vi "RunMacro_popup.vi"(0 "load?":bool, 1 "platform":u16(ring) items=["Mac", "PC"], 2 "command in":string, 3 "error in (no error)":errorcluster) -> (8 "Cancel":bool, 9 "command out":string, 10 "error out":errorcluster)   [LabVIEW 2020]
doc: "Sequence Program with the Message Handling Queue (MHQ) for the National High Magnetic Field Laboratory in Tallahassee, Florida. \nOnce you understand how the programs works, you should be able to modify this program easily. If you have any questions, contact Minseong Lee(ml10k@my.fsu.edu), who first made this program in June, 2015."
uses:
  <vilib>/Utility/file.llb/Read From Spreadsheet File (string).vi
panel:
  in  "Cancel button":bool
  in  "OK Button 2":bool
  in  "Cancel Button":bool
  in  "OK Button":bool
  out "Buffer Edit":string[](array[string])=["Wait for 1 s", "Wait for 2 s", "Wait for 1.1 s", "Wait for 1.2 s"]
  out "Path":path=path "C:/Users/shared/Sequences/MPMS_LCR_Tsweep.vi.txt"
  out "Buffer History":string[](array[string])
  in  "New Button":bool caption="New"
  in  "Commands":string(tree)="Wait for"
  in  "Sequence":i32[](listbox)=[4]
  in  "Save Button":bool caption="Save"
  in  "Save As Button":bool caption="Save As"
  out "Cursor Position":i32=4
  in  "Open Button":bool caption="Open"
  # "(1) Make a new or edit an existing sequence\n(2) Sequence must be saved\nNesting is allowed."
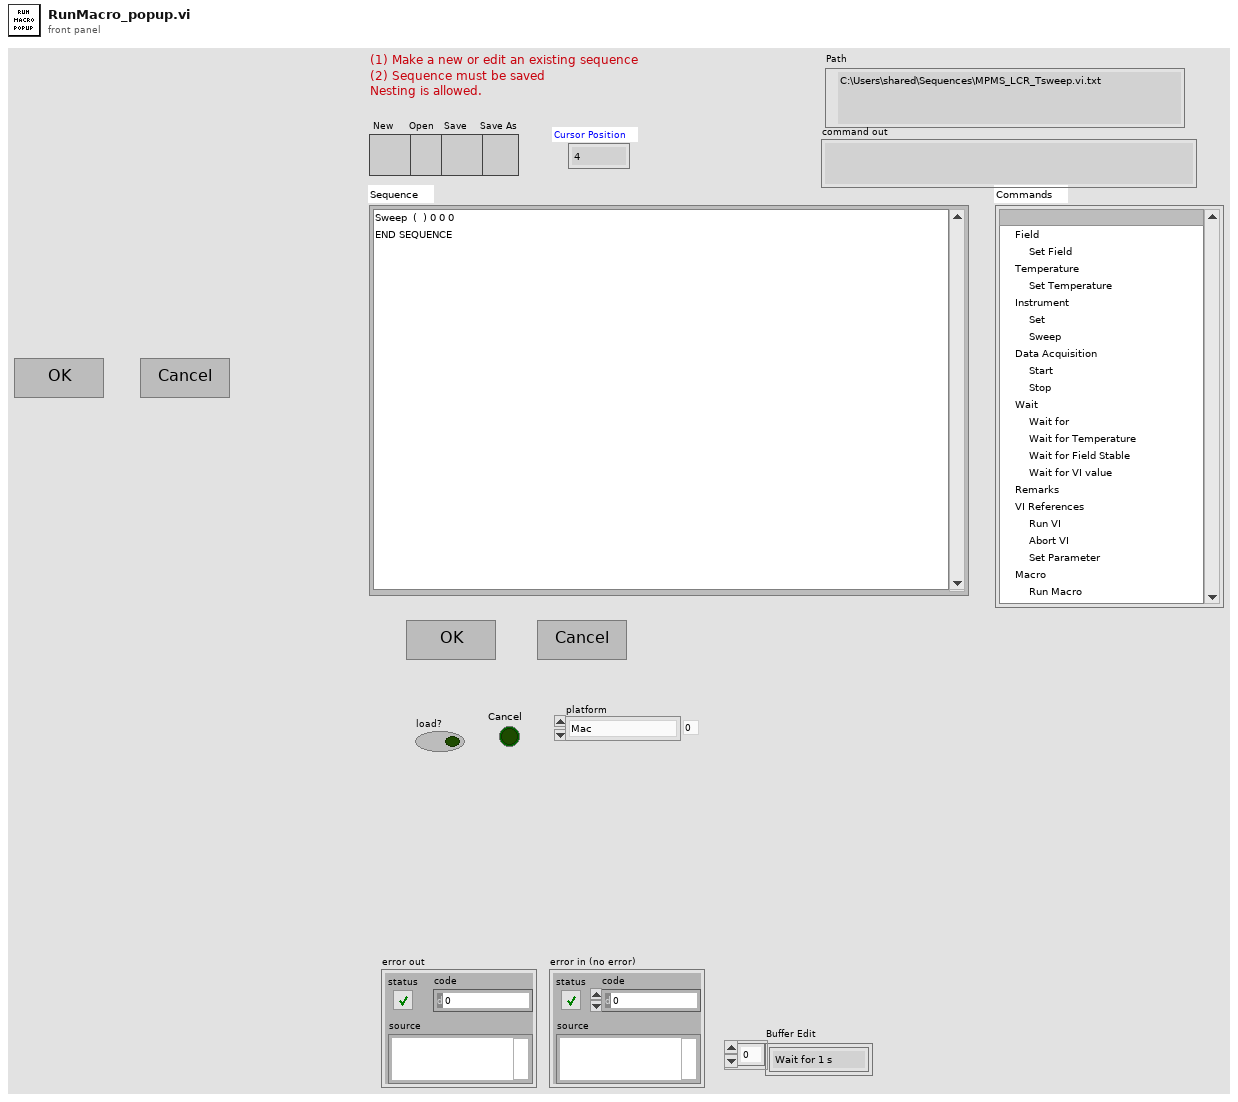
[diagram p1: front panel]
types:
  T1 = cluster{"No. of command":i32, "Parameters":string[], "Address":refnum<visa-resource-name>, "Boolean":bool, "No. of line":i32, "Initial Time":timestamp, "Current Time":timestamp, "Sequence status":string, "Sequence":refnum<vi>, "Temp_Check":i32, "Sequence_History":string, "Subsequence":string[]}
  T2 = cluster{"number of line":i32, "Signal":bool, "Command":string, "Sequence Reference":refnum<vi>, "Add or modification":bool}
  T3 = typedef "Command_Message.ctl" = cluster{"No. of command":i32, "Parameters":string[], "Address":refnum<visa-resource-name>, "Boolean":bool, "No. of line":i32, "Initial Time":timestamp, "Current Time":timestamp, "Status":string, "Sequence Ref.":refnum<vi>, "Temp check":i32, "Sequence_History":string, "Subsequence":string[]}
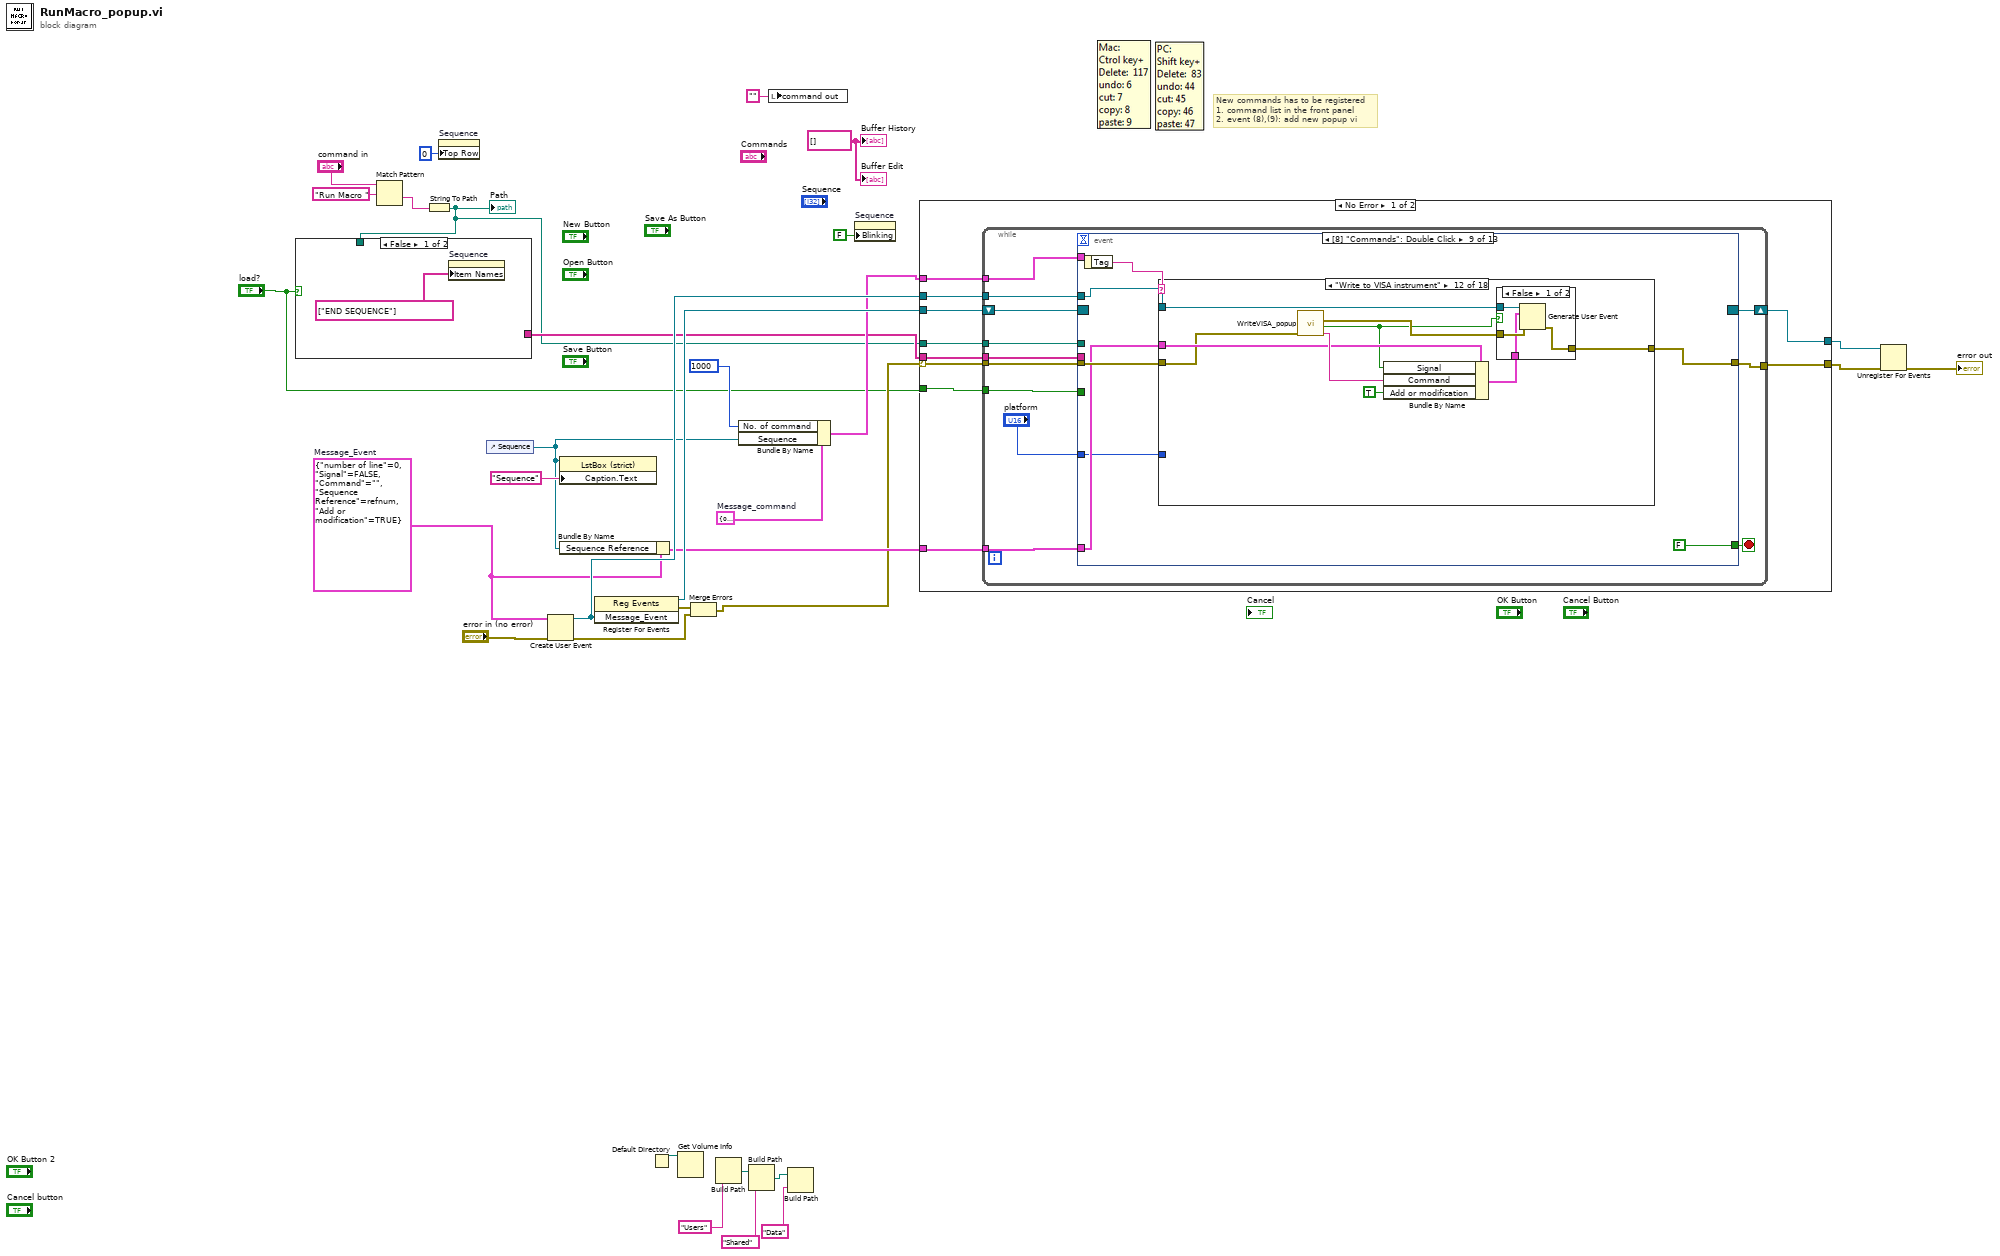
[diagram p0: block diagram]
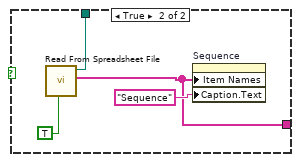
[diagram p2: hidden frame]
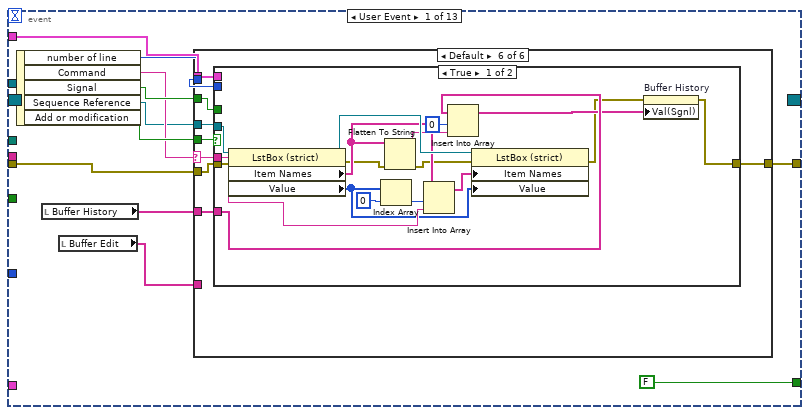
[diagram p3: hidden frame]
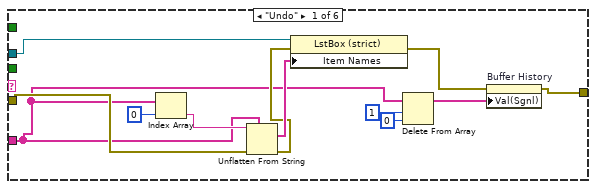
[diagram p4: hidden frame]
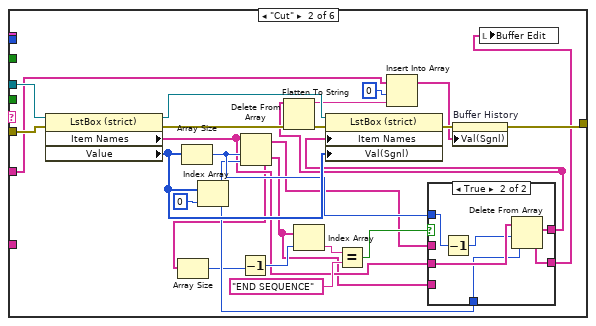
[diagram p5: hidden frame]
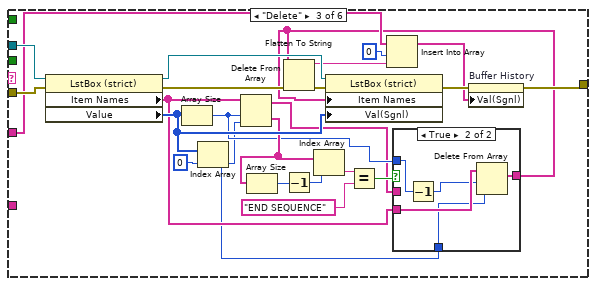
[diagram p7: hidden frame]
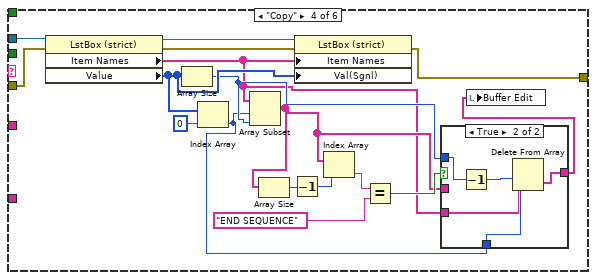
[diagram p9: hidden frame]
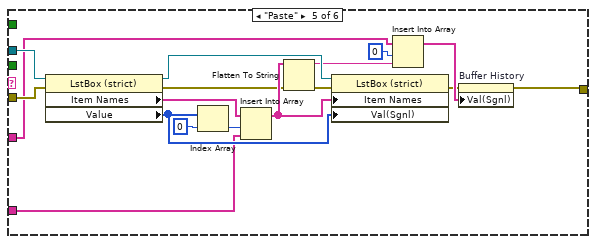
[diagram p11: hidden frame]
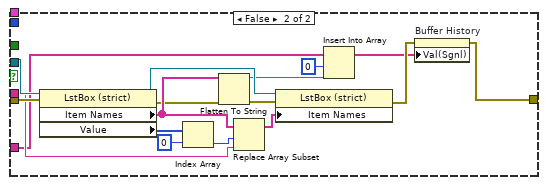
[diagram p12: hidden frame]
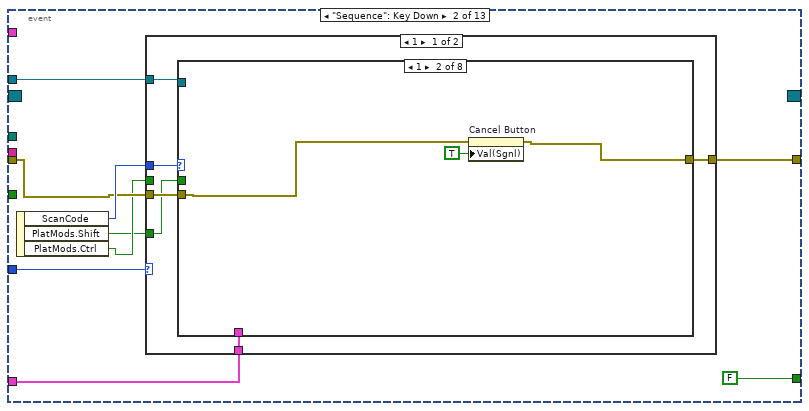
[diagram p13: hidden frame]
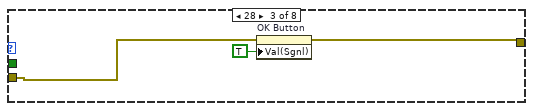
[diagram p15: hidden frame]
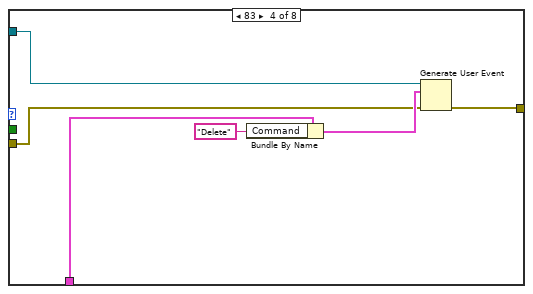
[diagram p16: hidden frame]
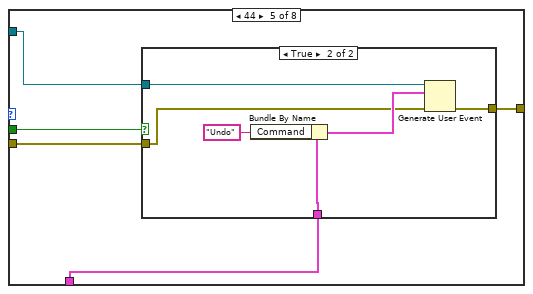
[diagram p17: hidden frame]
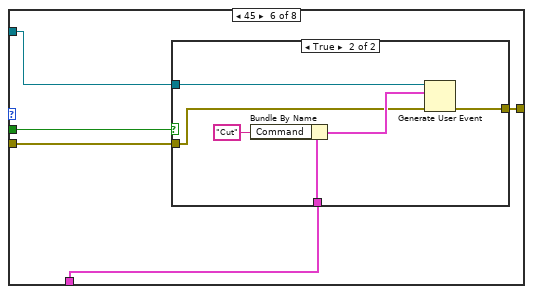
[diagram p19: hidden frame]
diagram:
  w10 = T1 {"No. of command"=0, "Parameters"=[], "Address"="", "Boolean"=TRUE, "No. of line"=0, "Initial Time"=timestamp(0 s since 1904-01-01), "Current Time"=timestamp(0 s since 1904-01-01), "Sequence status"="", "Sequence"=refnum, "Temp_Check"=0, "Sequence_History"="", "Subsequence"=[]}  # Message_command
  w20 = string[] []
  w25 = T2 {"number of line"=0, "Signal"=FALSE, "Command"="", "Sequence Reference"=refnum, "Add or modification"=TRUE}  # Message_Event
  # "New commands has to be registered\n1. command list in the front panel\n2. event (8),(9): add new popup vi"
  n1 = Match Pattern(string="command in", regular expression="Run Macro ") -> (after substring=w6:string)  [unwired: 1 in, 3 out]
  n2 = String To Path(string=w6) -> (path=w1:path)
  "Path" <- w1
  n3 = case shown="False" "load?" {
    tunnel: w1 -> [_ w36]
    tunnel: [_ w34] -> w5
    frame False {
      n4 = property on="Sequence" class="LstBox (strict)"("Item Names"=string[] ["END SEQUENCE"]) -> ()  [unwired: 2 in, 2 out]
    }
    frame True {
      n5 = call-poly <vilib>:"Read From Spreadsheet File.vi"("transpose (no:F)"=TRUE, "file path (dialog if empty)"=w36) -> ("first row"=w34:string[])  [unwired: 5 in, 4 out]
      n6 = property on="Sequence" class="LstBox (strict)"("Item Names"=w34, "Caption.Text"="Sequence") -> ()  [unwired: 2 in, 2 out]
    }
  }
  n7 = property on="Sequence" class="LstBox (strict)"("Top Row"=0) -> ()  [unwired: 2 in, 2 out]
  n8 = control-ref of="Sequence"() -> (w21:refnum<vi>)
  n9 = Create User Event(user event datatype=w25, error in="error in (no error)") -> (user event=w28:refnum<user-event>, error out=w30:errorcluster)
  n10 = property class="LstBox (strict)"(reference=w21, "Caption.Text"="Sequence") -> ()  [unwired: 1 in, 2 out]
  n11 = Bundle By Name(cluster=w25, "Sequence Reference"=w21) -> (w24:T2)
  n12 = register-events(w28) -> (reference out=w32:refnum<event-registration>, error out=w29:errorcluster)  [unwired: 2 in]
  n13 = Default Directory() -> (w13:path)
  n14 = Get Volume Info(11:w13) -> ()  [unwired: 1 in, 6 out]
  n15 = Merge Errors(w29, w30) -> (w12:errorcluster)
  n16 = Build Path(name or relative path="Users") -> (appended path=w16:path)  [unwired: 1 in]
  n17 = Bundle By Name(cluster=w10, "No. of command"=1000, "Sequence"=w21) -> (w9:T1)
  n18 = Build Path(base path=w16, name or relative path="Shared") -> (appended path=w15:path)
  n19 = local write "command out"("" ("command out")) -> ()
  n20 = Build Path(base path=w15, name or relative path="Data") -> ()  [unwired: 1 out]
  n21 = property on="Sequence" class="LstBox (strict)"("Blinking"=FALSE) -> ()  [unwired: 2 in, 2 out]
  n22 = case shown="No Error" w12 {
    selector: w12 -> [w46 w969]
    tunnel: [w41 w969] -> w26
    tunnel: w28 -> [w45 _]
    tunnel: w32 -> [w47 w968]
    tunnel: w9 -> [w44 _]
    tunnel: [w43 w968] -> w27
    tunnel: w24 -> [w42 _]
    tunnel: w1 -> [w40 _]
    tunnel: w5 -> [w39 _]
    tunnel: "load?" -> [w38 _]
    frame No Error {
      n23 = while {
        tunnel: w45 -> [w57]
        tunnel: w46 -> [w56]
        tunnel: [w55] -> w41
        tunnel: w44 -> [w54]
        shift-right: [w53] -> w43
        shift-left: w47 -> [w59]
        tunnel: w42 -> [w52]
        tunnel: w40 -> [w51]
        tunnel: w39 -> [w50]
        tunnel: w38 -> [w49]
        stop <- w58 stop-if-true
        # "Event_Handler"
        n24 = event shown="[8] \"Commands\": Double Click" {
          selector: w59 -> [_ _ _ _ _ _ _ _ _ _ _ _ _]
          dyn-events: [_ _ _ _ _ _ _ _ _ _ _ _ _] -> w53
          timeout: _ -> [_ _ _ _ _ _ _ _ _ _ _ _ _]
          tunnel: [FALSE ("NewVal") FALSE ("NewVal") FALSE ("NewVal") FALSE ("NewVal") FALSE ("NewVal") FALSE ("NewVal") FALSE ("NewVal") FALSE ("NewVal") FALSE ("NewVal") FALSE ("NewVal") FALSE ("NewVal") TRUE ("NewVal") TRUE ("NewVal")] -> w58
          tunnel: w57 -> [_ w234 w377 _ _ _ _ _ w542 w796 _ _ _]
          tunnel: w56 -> [w70 w235 w379 w409 w447 w461 w489 w516 w545 w805 w922 w929 w950]
          tunnel: [w69 w233 w378 w408 w445 w460 w488 w515 w543 w792 w922 w945 w955] -> w55
          tunnel: w54 -> [w68 _ _ _ _ _ _ _ _ w807 _ _ _]
          tunnel: w52 -> [_ w236 w376 _ _ _ _ _ w541 w797 _ _ _]
          tunnel: w51 -> [_ _ _ _ _ _ _ _ _ _ _ _ w952]
          tunnel: w50 -> [_ _ _ _ _ _ _ _ _ _ _ _ w951]
          tunnel: w49 -> [_ _ _ _ _ _ _ _ _ _ _ _ w953]
          tunnel: "platform" -> [_ w229 _ _ _ _ _ _ w539 w785 _ _ _]
          event User Event {
            n25 = event-data() -> ("number of line"=w67:i32, "Command"=w62:string, "Signal"=w65:bool, "Sequence Reference"=w60:refnum<vi>, "Add or modification"=w64:bool)  [unwired: 1 in]
            n26 = local read "Buffer History"() -> (w63:string[])
            n27 = local read "Buffer Edit"() -> (w61:string[])
            n28 = case shown="Default" w62 {
              selector: w62 -> [_ _ _ _ _ w186]
              tunnel: w70 -> [w74 w106 w138 w161 w184 w194]
              tunnel: [w72 w96 w128 w156 w169 w193] -> w69
              tunnel: w68 -> [_ _ _ _ _ w192]
              tunnel: w67 -> [_ _ _ _ _ w191]
              tunnel: w65 -> [_ _ _ _ _ w190]
              tunnel: w60 -> [w71 w107 w139 w162 w185 w189]
              tunnel: w64 -> [_ _ _ _ _ w188]
              tunnel: w63 -> [w73 w101 w133 _ w175 w187]
              tunnel: w61 -> [_ _ _ _ w178 _]
              frame "Undo" {
                n29 = Index Array(array=w73, index=0) -> (element=w81:string)
                n30 = Unflatten From String(type=w73, binary string=w81, error in (no error)=w74) -> (value=w80:string[], error out=w79:errorcluster)  [unwired: 2 in, 1 out]
                n31 = property on="Property Node" class="LstBox (strict)"(reference=w71, error in=w79, "Item Names"=w80) -> (error out=w75:errorcluster)  [unwired: 1 out]
                n32 = Delete From Array(array=w73, length=1, index=0) -> (array with subset deleted=w76:string[])  [unwired: 1 out]
                n33 = property on="Buffer History" class="Arr (strict)"(error in=w75, "Val(Sgnl)"=w76) -> (error out=w72:errorcluster)  [unwired: 1 in, 1 out]
              }
              frame "Cut" {
                n34 = property on="Property Node" class="LstBox (strict)"(reference=w107, error in=w106) -> (reference out=w104:refnum<vi>, error out=w102:errorcluster, "Item Names"=w86:string[], "Value"=w103:i32[])
                n35 = Array Size(array=w103) -> (size(s)=w94:i32)
                n36 = Index Array(array=w103, index=0) -> (element=w93:i32)
                n37 = Delete From Array(array=w86, length=w94, index=w93) -> (deleted portion=w84:string[], array with subset deleted=w87:string[])
                n38 = Array Size(array=w84) -> (size(s)=w92:i32)
                n39 = Decrement(x=w92) -> (x-1=w91:i32)
                n40 = Index Array(array=w84, index=w91) -> (element=w89:string)
                n41 = Equal?(x=w89, y="END SEQUENCE") -> (x = y?=w88:bool)
                n42 = case shown="True" w88 {
                  tunnel: w86 -> [_ w115]
                  tunnel: w94 -> [_ w114]
                  tunnel: w93 -> [_ w112]
                  tunnel: [w109 w111] -> w85
                  tunnel: w87 -> [w109 _]
                  tunnel: w84 -> [w108 _]
                  tunnel: [w108 w110] -> w83
                  frame False {
                  }
                  frame True {
                    n43 = Decrement(x=w114) -> (x-1=w113:i32)
                    n44 = Delete From Array(array=w115, length=w113, index=w112) -> (deleted portion=w110:string[], array with subset deleted=w111:string[])
                  }
                }
                n45 = Flatten To String(anything=w85, error in (no error)=w102) -> (data string=w99:string, error out=w98:errorcluster)  [unwired: 2 in, 1 out]
                n46 = property on="Property Node" class="LstBox (strict)"(reference=w104, error in=w98, "Item Names"=w85, "Val(Sgnl)"=w103) -> (error out=w97:errorcluster)  [unwired: 1 out]
                n47 = Insert Into Array(array=w101, index=0, new element=w99) -> (w95:string[])
                n48 = property on="Buffer History" class="Arr (strict)"(error in=w97, "Val(Sgnl)"=w95) -> (error out=w96:errorcluster)  [unwired: 1 in, 1 out]
                n49 = local write "Buffer Edit"(w83) -> ()
              }
              frame "Delete" {
                n50 = property on="Property Node" class="LstBox (strict)"(reference=w139, error in=w138) -> (reference out=w136:refnum<vi>, error out=w134:errorcluster, "Item Names"=w120:string[], "Value"=w135:i32[])
                n51 = Array Size(array=w135) -> (size(s)=w119:i32)
                n52 = Index Array(array=w135, index=0) -> (element=w118:i32)
                n53 = Delete From Array(array=w120, length=w119, index=w118) -> (deleted portion=w126:string[], array with subset deleted=w117:string[])
                n54 = Array Size(array=w126) -> (size(s)=w122:i32)
                n55 = Decrement(x=w122) -> (x-1=w121:i32)
                n56 = Index Array(array=w126, index=w121) -> (element=w125:string)
                n57 = Equal?(x=w125, y="END SEQUENCE") -> (x = y?=w123:bool)
                n58 = case shown="True" w123 {
                  tunnel: w120 -> [_ w145]
                  tunnel: w119 -> [_ w144]
                  tunnel: w118 -> [_ w142]
                  tunnel: [w140 w141] -> w116
                  tunnel: w117 -> [w140 _]
                  frame False {
                  }
                  frame True {
                    n59 = Decrement(x=w144) -> (x-1=w143:i32)
                    n60 = Delete From Array(array=w145, length=w143, index=w142) -> (array with subset deleted=w141:string[])  [unwired: 1 out]
                  }
                }
                n61 = Flatten To String(anything=w116, error in (no error)=w134) -> (data string=w131:string, error out=w130:errorcluster)  [unwired: 2 in, 1 out]
                n62 = property on="Property Node" class="LstBox (strict)"(reference=w136, error in=w130, "Item Names"=w116, "Val(Sgnl)"=w135) -> (error out=w129:errorcluster)  [unwired: 1 out]
                n63 = Insert Into Array(array=w133, index=0, new element=w131) -> (w127:string[])
                n64 = property on="Buffer History" class="Arr (strict)"(error in=w129, "Val(Sgnl)"=w127) -> (error out=w128:errorcluster)  [unwired: 1 in, 1 out]
              }
              frame "Copy" {
                n65 = property on="Property Node" class="LstBox (strict)"(reference=w162, error in=w161) -> (reference out=w159:refnum<vi>, error out=w158:errorcluster, "Item Names"=w146:string[], "Value"=w157:i32[])
                n66 = Array Size(array=w157) -> (size(s)=w150:i32)
                n67 = Index Array(array=w157, index=0) -> (element=w149:i32)
                n68 = Array Subset(array=w146, index=w149, length=w150) -> (w148:string[])
                n69 = Array Size(array=w148) -> (size(s)=w155:i32)
                n70 = Decrement(x=w155) -> (x-1=w154:i32)
                n71 = property on="Property Node" class="LstBox (strict)"(reference=w159, error in=w158, "Item Names"=w146, "Val(Sgnl)"=w157) -> (error out=w156:errorcluster)  [unwired: 1 out]
                n72 = Index Array(array=w148, index=w154) -> (element=w153:string)
                n73 = Equal?(x=w153, y="END SEQUENCE") -> (x = y?=w151:bool)
                n74 = case shown="True" w151 {
                  tunnel: w150 -> [_ w168]
                  tunnel: w149 -> [_ w166]
                  tunnel: [w163 w164] -> w147
                  tunnel: w148 -> [w163 _]
                  tunnel: w146 -> [_ w165]
                  frame False {
                  }
                  frame True {
                    n75 = Decrement(x=w168) -> (x-1=w167:i32)
                    n76 = Delete From Array(array=w165, length=w167, index=w166) -> (deleted portion=w164:string[])  [unwired: 1 out]
                  }
                }
                n77 = local write "Buffer Edit"(w147) -> ()
              }
              frame "Paste" {
                n78 = property on="Property Node" class="LstBox (strict)"(reference=w185, error in=w184) -> (reference out=w182:refnum<vi>, error out=w172:errorcluster, "Item Names"=w179:string[], "Value"=w181:i32[])
                n79 = Index Array(array=w181, index=0) -> (element=w180:i32)
                n80 = Insert Into Array(array=w179, index=w180, new element=w178) -> (w176:string[])
                n81 = Flatten To String(anything=w176, error in (no error)=w172) -> (data string=w177:string, error out=w171:errorcluster)  [unwired: 2 in, 1 out]
                n82 = property on="Property Node" class="LstBox (strict)"(reference=w182, error in=w171, "Item Names"=w176, "Val(Sgnl)"=w181) -> (error out=w170:errorcluster)  [unwired: 1 out]
                n83 = Insert Into Array(array=w175, index=0, new element=w177) -> (w173:string[])
                n84 = property on="Buffer History" class="Arr (strict)"(error in=w170, "Val(Sgnl)"=w173) -> (error out=w169:errorcluster)  [unwired: 1 in, 1 out]
              }
              frame Default {
                n85 = case shown="True" w188 {
                  tunnel: w194 -> [w211 w228]
                  tunnel: [w195 w212] -> w193
                  tunnel: w192 -> [_ _]
                  tunnel: w191 -> [_ _]
                  tunnel: w190 -> [_ _]
                  tunnel: w189 -> [w210 w227]
                  tunnel: w186 -> [w209 w226]
                  tunnel: w187 -> [w208 w225]
                  frame True {
                    n86 = property class="LstBox (strict)"(reference=w210, error in=w211) -> (reference out=w205:refnum<vi>, error out=w199:errorcluster, "Item Names"=w201:string[], "Value"=w204:i32[])
                    n87 = Index Array(array=w204, index=0) -> (element=w206:i32)
                    n88 = Flatten To String(anything=w201, error in (no error)=w199) -> (data string=w202:string, error out=w200:errorcluster)  [unwired: 2 in, 1 out]
                    n89 = Insert Into Array(array=w201, index=w206, new element=w209) -> (w203:string[])
                    n90 = Insert Into Array(array=w208, index=0, new element=w202) -> (w197:string[])
                    n91 = property class="LstBox (strict)"(reference=w205, error in=w200, "Item Names"=w203, "Value"=w204) -> (error out=w196:errorcluster)  [unwired: 1 out]
                    n92 = property on="Buffer History" class="Arr (strict)"(error in=w196, "Val(Sgnl)"=w197) -> (error out=w195:errorcluster)  [unwired: 1 in, 1 out]
                  }
                  frame False {
                    n93 = property class="LstBox (strict)"(reference=w227, error in=w228) -> (reference out=w222:refnum<vi>, error out=w217:errorcluster, "Item Names"=w218:string[], "Value"=w221:i32[])
                    n94 = Index Array(array=w221, index=0) -> (element=w223:i32)
                    n95 = Flatten To String(anything=w218, error in (no error)=w217) -> (data string=w220:string, error out=w216:errorcluster)  [unwired: 2 in, 1 out]
                    n96 = Replace Array Subset(array=w218, new element=w226, index=w223) -> (w219:string[])
                    n97 = property class="LstBox (strict)"(reference=w222, error in=w216, "Item Names"=w219) -> (error out=w214:errorcluster)  [unwired: 1 out]
                    n98 = Insert Into Array(array=w225, index=0, new element=w220) -> (w213:string[])
                    n99 = property on="Buffer History" class="Arr (strict)"(error in=w214, "Val(Sgnl)"=w213) -> (error out=w212:errorcluster)  [unwired: 1 in, 1 out]
                  }
                }
              }
            }
          }
          event "Sequence": Key Down {
            n100 = event-data() -> ("ScanCode"=w237:i16, "PlatMods.Shift"=w230:bool, "PlatMods.Ctrl"=w231:bool)  [unwired: 1 in]
            n101 = case shown="1" w229 {
              tunnel: w237 -> [w243 w310]
              tunnel: w236 -> [w242 w309]
              tunnel: w235 -> [w241 w308]
              tunnel: w234 -> [w240 w307]
              tunnel: [w239 w306] -> w233
              tunnel: w231 -> [_ w305]
              tunnel: w230 -> [w238 _]
              frame 1 {
                n102 = case shown="1" w243 {
                  tunnel: w242 -> [_ _ _ w255 w258 w270 w282 w294]
                  tunnel: w241 -> [w244 w246 w249 w253 w260 w272 w284 w296]
                  tunnel: w240 -> [_ _ _ w252 w257 w269 w281 w293]
                  tunnel: [w244 w245 w248 w251 w259 w271 w283 w295] -> w239
                  tunnel: w238 -> [_ _ _ _ w261 w273 w285 w297]
                  frame 0, Default {
                  }
                  frame 1 {
                    n103 = property on="Cancel Button" class="Bool (strict)"(error in=w246, "Val(Sgnl)"=TRUE ("Value (Signaling)")) -> (error out=w245:errorcluster)  [unwired: 1 in, 1 out]
                  }
                  frame 28 {
                    n104 = property on="OK Button" class="Bool (strict)"(error in=w249, "Val(Sgnl)"=TRUE ("Value (Signaling)")) -> (error out=w248:errorcluster)  [unwired: 1 in, 1 out]
                  }
                  frame 83 {
                    n105 = Bundle By Name(cluster=w255, "Command"="Delete") -> (w254:T2)
                    n106 = Generate User Event(user event=w252, event data cluster=w254, error in=w253) -> (error out=w251:errorcluster)  [unwired: 1 in, 1 out]
                  }
                  frame 44 {
                    n107 = case shown="True" w261 {
                      tunnel: w260 -> [w262 w264]
                      tunnel: [w262 w266] -> w259
                      tunnel: w258 -> [_ w265]
                      tunnel: w257 -> [_ w263]
                      frame False {
                      }
                      frame True {
                        n108 = Bundle By Name(cluster=w265, "Command"="Undo") -> (w267:T2)
                        n109 = Generate User Event(user event=w263, event data cluster=w267, error in=w264) -> (error out=w266:errorcluster)  [unwired: 1 in, 1 out]
                      }
                    }
                  }
                  frame 45 {
                    n110 = case shown="True" w273 {
                      tunnel: w272 -> [w274 w276]
                      tunnel: [w274 w278] -> w271
                      tunnel: w270 -> [_ w277]
                      tunnel: w269 -> [_ w275]
                      frame False {
                      }
                      frame True {
                        n111 = Bundle By Name(cluster=w277, "Command"="Cut") -> (w279:T2)
                        n112 = Generate User Event(user event=w275, event data cluster=w279, error in=w276) -> (error out=w278:errorcluster)  [unwired: 1 in, 1 out]
                      }
                    }
                  }
                  frame 46 {
                    n113 = case shown="True" w285 {
                      tunnel: w284 -> [w286 w288]
                      tunnel: [w286 w290] -> w283
                      tunnel: w282 -> [_ w289]
                      tunnel: w281 -> [_ w287]
                      frame False {
                      }
                      frame True {
                        n114 = Bundle By Name(cluster=w289, "Command"="Copy") -> (w291:T2)
                        n115 = Generate User Event(user event=w287, event data cluster=w291, error in=w288) -> (error out=w290:errorcluster)  [unwired: 1 in, 1 out]
                      }
                    }
                  }
                  frame 47 {
                    n116 = case shown="False" w297 {
                      tunnel: w296 -> [w298 w300]
                      tunnel: [w298 w302] -> w295
                      tunnel: w294 -> [_ w301]
                      tunnel: w293 -> [_ w299]
                      frame False {
                      }
                      frame True {
                        n117 = Bundle By Name(cluster=w301, "Command"="Paste") -> (w303:T2)
                        n118 = Generate User Event(user event=w299, event data cluster=w303, error in=w300) -> (error out=w302:errorcluster)  [unwired: 1 in, 1 out]
                      }
                    }
                  }
                }
              }
              frame 0, Default {
                n119 = case shown="36" w310 {
                  tunnel: w309 -> [_ _ _ _ w325 w328 w340 w352 w364]
                  tunnel: w308 -> [w311 w313 w316 w319 w323 w330 w342 w354 w366]
                  tunnel: w307 -> [_ _ _ _ w322 w327 w339 w351 w363]
                  tunnel: [w311 w312 w315 w318 w321 w329 w341 w353 w365] -> w306
                  tunnel: w305 -> [_ _ _ _ _ w331 w343 w355 w367]
                  frame 0, Default {
                  }
                  frame 36 {
                    n120 = property on="OK Button" class="Bool (strict)"(error in=w313, "Val(Sgnl)"=TRUE ("Value (Signaling)")) -> (error out=w312:errorcluster)  [unwired: 1 in, 1 out]
                  }
                  frame 76 {
                    n121 = property on="OK Button" class="Bool (strict)"(error in=w316, "Val(Sgnl)"=TRUE ("Value (Signaling)")) -> (error out=w315:errorcluster)  [unwired: 1 in, 1 out]
                  }
                  frame 53 {
                    n122 = property on="Cancel Button" class="Bool (strict)"(error in=w319, "Val(Sgnl)"=TRUE ("Value (Signaling)")) -> (error out=w318:errorcluster)  [unwired: 1 in, 1 out]
                  }
                  frame 117 {
                    n123 = Bundle By Name(cluster=w325, "Command"="Delete") -> (w324:T2)
                    n124 = Generate User Event(user event=w322, event data cluster=w324, error in=w323) -> (error out=w321:errorcluster)  [unwired: 1 in, 1 out]
                  }
                  frame 6 {
                    n125 = case shown="True" w331 {
                      tunnel: w330 -> [w332 w334]
                      tunnel: [w332 w336] -> w329
                      tunnel: w328 -> [_ w335]
                      tunnel: w327 -> [_ w333]
                      frame False {
                      }
                      frame True {
                        n126 = Bundle By Name(cluster=w335, "Command"="Undo") -> (w337:T2)
                        n127 = Generate User Event(user event=w333, event data cluster=w337, error in=w334) -> (error out=w336:errorcluster)  [unwired: 1 in, 1 out]
                      }
                    }
                  }
                  frame 7 {
                    n128 = case shown="True" w343 {
                      tunnel: w342 -> [w344 w346]
                      tunnel: [w344 w348] -> w341
                      tunnel: w340 -> [_ w347]
                      tunnel: w339 -> [_ w345]
                      frame False {
                      }
                      frame True {
                        n129 = Bundle By Name(cluster=w347, "Command"="Cut") -> (w349:T2)
                        n130 = Generate User Event(user event=w345, event data cluster=w349, error in=w346) -> (error out=w348:errorcluster)  [unwired: 1 in, 1 out]
                      }
                    }
                  }
                  frame 8 {
                    n131 = case shown="True" w355 {
                      tunnel: w354 -> [w356 w358]
                      tunnel: [w356 w360] -> w353
                      tunnel: w352 -> [_ w359]
                      tunnel: w351 -> [_ w357]
                      frame False {
                      }
                      frame True {
                        n132 = Bundle By Name(cluster=w359, "Command"="Copy") -> (w361:T2)
                        n133 = Generate User Event(user event=w357, event data cluster=w361, error in=w358) -> (error out=w360:errorcluster)  [unwired: 1 in, 1 out]
                      }
                    }
                  }
                  frame 9 {
                    n134 = case shown="False" w367 {
                      tunnel: w366 -> [w368 w370]
                      tunnel: [w368 w372] -> w365
                      tunnel: w364 -> [_ w371]
                      tunnel: w363 -> [_ w369]
                      frame False {
                      }
                      frame True {
                        n135 = Bundle By Name(cluster=w371, "Command"="Paste") -> (w373:T2)
                        n136 = Generate User Event(user event=w369, event data cluster=w373, error in=w370) -> (error out=w372:errorcluster)  [unwired: 1 in, 1 out]
                      }
                    }
                  }
                }
              }
            }
          }
          event "Sequence": Shortcut Menu Selection (User) {
            n137 = event-data() -> ("ItemTag"=w380:string)  [unwired: 1 in]
            n138 = case shown="\"Paste\"" w380 {
              selector: w380 -> [_ w385 w391 w397 w403]
              tunnel: w379 -> [w381 w383 w389 w395 w401]
              tunnel: [w381 w382 w388 w394 w400] -> w378
              tunnel: w377 -> [_ w387 w393 w399 w405]
              tunnel: w376 -> [_ w386 w392 w398 w404]
              frame Default {
              }
              frame "Undo" {
                n139 = Bundle By Name(cluster=w386, "Command"=w385) -> (w384:T2)
                n140 = Generate User Event(user event=w387, event data cluster=w384, error in=w383) -> (error out=w382:errorcluster)  [unwired: 1 in, 1 out]
              }
              frame "Cut" {
                n141 = Bundle By Name(cluster=w392, "Command"=w391) -> (w390:T2)
                n142 = Generate User Event(user event=w393, event data cluster=w390, error in=w389) -> (error out=w388:errorcluster)  [unwired: 1 in, 1 out]
              }
              frame "Copy" {
                n143 = Bundle By Name(cluster=w398, "Command"=w397) -> (w396:T2)
                n144 = Generate User Event(user event=w399, event data cluster=w396, error in=w395) -> (error out=w394:errorcluster)  [unwired: 1 in, 1 out]
              }
              frame "Paste" {
                n145 = Bundle By Name(cluster=w404, "Command"=w403) -> (w402:T2)
                n146 = Generate User Event(user event=w405, event data cluster=w402, error in=w401) -> (error out=w400:errorcluster)  [unwired: 1 in, 1 out]
              }
            }
          }
          event "New Button": Value Change {
            n147 = event-data() -> ("NewVal"=w410:bool, "CtlRef"=w407:refnum<vi>)  [unwired: 1 in]
            n148 = case shown="True" w410 {
              tunnel: w409 -> [w411 w427]
              tunnel: [w411 w419] -> w408
              tunnel: w407 -> [_ w422]
              frame False {
              }
              frame True {
                n149 = property on="Sequence" class="LstBox (strict)"(error in=w427) -> (error out=w418:errorcluster, "Caption.Text"=w426:string, "Item Names"=w423:string[])  [unwired: 1 in, 1 out]
                n150 = property on="Buffer History" class="Arr (strict)"(error in=w418) -> (error out=w417:errorcluster, "Value"=w416:string[])  [unwired: 1 in, 1 out]
                n151 = Equal?(x=w426, y="Sequence*") -> (x = y?=w424:bool)
                n152 = case shown="False" w424 {
                  tunnel: w417 -> [w432 w443]
                  tunnel: w423 -> [_ w444]
                  tunnel: [w433 w438] -> w415
                  tunnel: w422 -> [w431 w437]
                  tunnel: [w431 w437] -> w421
                  tunnel: w416 -> [_ w435]
                  tunnel: [string[] [] ("Buffer out") w434] -> w413
                  frame False {
                    n153 = property on="Sequence" class="LstBox (strict)"(error in=w432, "Item Names"=string[] ["END SEQUENCE"], "Caption.Text"="Sequence") -> (error out=w433:errorcluster)  [unwired: 1 in, 1 out]
                  }
                  frame True {
                    n154 = property on="Path" class="Path"(error in=w443) -> (error out=w442:errorcluster, "Value"=w441:path)  [unwired: 1 in, 1 out]
                    n155 = call "New_File.vi"("error in (no error)"=w442, "Path"=w441, "Buffer in"=w435, "Sequence in"=w444) -> ("error out"=w440:errorcluster, "Sequence Caption"=w436:string, "Buffer out"=w434:string[], "Sequence_out"=w439:string[])  [unwired: 4 in]
                    n156 = property on="Sequence" class="LstBox (strict)"(error in=w440, "Item Names"=w439, "Caption.Text"=w436) -> (error out=w438:errorcluster)  [unwired: 1 in, 1 out]
                  }
                }
                n157 = property on="Buffer History" class="Arr (strict)"(error in=w415, "Value"=w413) -> (error out=w414:errorcluster)  [unwired: 1 in, 1 out]
                n158 = property class="Bool (strict)"(reference=w421, error in=w414, "Value"=FALSE) -> (error out=w419:errorcluster)  [unwired: 1 out]
                n159 = property on="Sequence" class="LstBox (strict)"("Top Row"=0) -> ()  [unwired: 2 in, 2 out]
              }
            }
          }
          event "Buffer History": Value Change {
            n160 = event-data() -> ("NewVal"=w451:string[])  [unwired: 1 in]
            n161 = Array Size(array=w451) -> (size(s)=w450:i32)
            n162 = Equal?(x=w450, y=0) -> (x = y?=w448:bool)
            n163 = case shown="False" w448 {
              tunnel: w447 -> [w453 w456]
              tunnel: [w452 w455] -> w445
              frame True {
                n164 = property on="Sequence" class="LstBox (strict)"(error in=w453, "Caption.Text"="Sequence") -> (error out=w452:errorcluster)  [unwired: 1 in, 1 out]
              }
              frame False {
                n165 = property on="Sequence" class="LstBox (strict)"(error in=w456, "Caption.Text"="Sequence*") -> (error out=w455:errorcluster)  [unwired: 1 in, 1 out]
              }
            }
          }
          event "Open Button": Value Change {
            n166 = event-data() -> ("NewVal"=w462:bool, "CtlRef"=w459:refnum<vi>)  [unwired: 1 in]
            n167 = case shown="True" w462 {
              tunnel: w461 -> [w463 w485]
              tunnel: [w463 w466] -> w460
              tunnel: w459 -> [_ w469]
              frame False {
              }
              frame True {
                n168 = property on="Sequence" class="LstBox (strict)"(error in=w485) -> (error out=w481:errorcluster, "Caption.Text"=w483:string, "Item Names"=w482:string[])  [unwired: 1 in, 1 out]
                n169 = Equal?(x=w483, y="Sequence*") -> (x = y?=w470:bool)
                n170 = property on="Buffer History" class="Arr (strict)"(error in=w481) -> (error out=w479:errorcluster, "Value"=w480:string[])  [unwired: 1 in, 1 out]
                n171 = property on="Path" class="Path"(error in=w479) -> (error out=w477:errorcluster, "Value"=w478:path)  [unwired: 1 in, 1 out]
                n172 = call "Open_File.vi"("Message?"=w470, "Path in"=w478, "error in (no error)"=w477, "Sequence in"=w482, "Buffer in"=w480, "Sequence Caption in"=w483) -> ("error out"=w465:errorcluster, "Sequence out"=w475:string[], "Buffer out"=w473:string[], "Sequence Caption out"=w476:string, "Path out"=w471:path, "top row"=w464:i32)
                n173 = property on="Sequence" class="LstBox (strict)"("Top Row"=w464) -> ()  [unwired: 2 in, 2 out]
                n174 = property on="Sequence" class="LstBox (strict)"(error in=w465, "Item Names"=w475, "Caption.Text"=w476) -> (error out=w474:errorcluster)  [unwired: 1 in, 1 out]
                n175 = property on="Buffer History" class="Arr (strict)"(error in=w474, "Value"=w473) -> (error out=w472:errorcluster)  [unwired: 1 in, 1 out]
                n176 = property on="Path" class="Path"(error in=w472, "Value"=w471) -> (error out=w468:errorcluster)  [unwired: 1 in, 1 out]
                n177 = property class="Bool (strict)"(reference=w469, error in=w468, "Value"=FALSE) -> (error out=w466:errorcluster)  [unwired: 1 out]
              }
            }
          }
          event "Save Button": Value Change {
            n178 = event-data() -> ("NewVal"=w490:bool, "CtlRef"=w487:refnum<vi>)  [unwired: 1 in]
            n179 = case shown="True" w490 {
              tunnel: w489 -> [w491 w508]
              tunnel: [w491 w492] -> w488
              tunnel: w487 -> [_ w495]
              frame False {
              }
              frame True {
                n180 = property on="Path" class="Path"(error in=w508) -> (error out=w507:errorcluster, "Value"=w510:path)  [unwired: 1 in, 1 out]
                n181 = Not Equal?(x=path "", y=w510) -> (x != y?=w511:bool)
                n182 = property on="Buffer History" class="Arr (strict)"(error in=w507) -> (error out=w506:errorcluster, "Value"=w509:string[])  [unwired: 1 in, 1 out]
                n183 = property on="Sequence" class="LstBox (strict)"(error in=w506) -> (error out=w505:errorcluster, "Item Names"=w504:string[], "Caption.Text"=w503:string)  [unwired: 1 in, 1 out]
                n184 = call "Save_File.vi"("Sequence caption in"=w503, "Path?"=w511, "error in (no error)"=w505, "Sequence in"=w504, "Buffer in"=w509, "Path in"=w510) -> ("error out"=w502:errorcluster, "Sequence out"=w498:string[], "Buffer out"=w500:string[], "Path out"=w496:path, "Sequence caption out"=w499:string)  [unwired: 1 in]
                n185 = property on="Buffer History" class="Arr (strict)"(error in=w502, "Value"=w500) -> (error out=w501:errorcluster)  [unwired: 1 in, 1 out]
                n186 = property on="Sequence" class="LstBox (strict)"(error in=w501, "Item Names"=w498, "Caption.Text"=w499) -> (error out=w497:errorcluster)  [unwired: 1 in, 1 out]
                n187 = property on="Path" class="Path"(error in=w497, "Value"=w496) -> (error out=w494:errorcluster)  [unwired: 1 in, 1 out]
                n188 = property class="Bool (strict)"(reference=w495, error in=w494, "Value"=FALSE) -> (error out=w492:errorcluster)  [unwired: 1 out]
              }
            }
          }
          event "Save As Button": Value Change {
            n189 = event-data() -> ("NewVal"=w517:bool, "CtlRef"=w514:refnum<vi>)  [unwired: 1 in]
            n190 = case shown="True" w517 {
              tunnel: w516 -> [w518 w536]
              tunnel: [w518 w520] -> w515
              tunnel: w514 -> [_ w523]
              frame False {
              }
              frame True {
                n191 = property on="Path" class="Path"(error in=w536) -> (error out=w535:errorcluster, "Value"=w538:path)  [unwired: 1 in, 1 out]
                n192 = property on="Buffer History" class="Arr (strict)"(error in=w535) -> (error out=w534:errorcluster, "Value"=w537:string[])  [unwired: 1 in, 1 out]
                n193 = property on="Sequence" class="LstBox (strict)"(error in=w534) -> (error out=w533:errorcluster, "Item Names"=w532:string[], "Caption.Text"=w531:string)  [unwired: 1 in, 1 out]
                n194 = call "Save_File.vi"("Sequence caption in"=w531, "Path?"=FALSE, "error in (no error)"=w533, "Sequence in"=w532, "Buffer in"=w537, "Path in"=w538) -> ("error out"=w530:errorcluster, "Sequence out"=w526:string[], "Buffer out"=w528:string[], "Path out"=w524:path, "Sequence caption out"=w527:string)  [unwired: 1 in]
                n195 = property on="Buffer History" class="Arr (strict)"(error in=w530, "Value"=w528) -> (error out=w529:errorcluster)  [unwired: 1 in, 1 out]
                n196 = property on="Sequence" class="LstBox (strict)"(error in=w529, "Item Names"=w526, "Caption.Text"=w527) -> (error out=w525:errorcluster)  [unwired: 1 in, 1 out]
                n197 = property on="Path" class="Path"(error in=w525, "Value"=w524) -> (error out=w522:errorcluster)  [unwired: 1 in, 1 out]
                n198 = property class="Bool (strict)"(reference=w523, error in=w522, "Value"=FALSE) -> (error out=w520:errorcluster)  [unwired: 1 out]
              }
            }
          }
          event "Commands": Double Click {
            n199 = event-data() -> ("Tag"=w544:string)  [unwired: 1 in]
            n200 = case shown="\"Write to VISA instrument\"" w544 {
              tunnel: w545 -> [w546 w549 w563 w577 w591 w605 w619 w633 w647 w661 w675 w689 w703 w717 w730 w744 w759 w775]
              tunnel: [w546 w551 w565 w579 w593 w607 w621 w635 w649 w663 w677 w691 w705 w719 w734 w748 w762 w778] -> w543
              tunnel: w542 -> [_ w555 w569 w583 w597 w611 w625 w639 w653 w667 w681 w695 w709 w723 w736 w749 w763 w779]
              tunnel: w541 -> [_ w550 w564 w578 w592 w606 w620 w634 w648 w662 w676 w690 w704 w718 w733 w747 w761 w777]
              tunnel: w539 -> [_ _ _ _ _ _ _ _ _ _ _ _ _ _ _ _ _ w769]
              frame Default {
              }
              frame "Set Field" {
                n201 = call "SetField_popup.vi"("error in (no error)"=w549) -> ("Output Line command"=w553:string, "Cancel"=w547:bool, "error out"=w554:errorcluster)  [unwired: 5 in]
                n202 = Bundle By Name(cluster=w550, "Signal"=w547, "Command"=w553, "Add or modification"=TRUE) -> (w552:T2)
                n203 = case shown="True" w547 {
                  tunnel: w555 -> [w559 _]
                  tunnel: w554 -> [w558 w560]
                  tunnel: w552 -> [w557 _]
                  tunnel: [w556 w560] -> w551
                  frame False {
                    n204 = Generate User Event(user event=w559, event data cluster=w557, error in=w558) -> (error out=w556:errorcluster)  [unwired: 1 in, 1 out]
                  }
                  frame True {
                  }
                }
              }
              frame "Set Temperature" {
                n205 = call "SetTemp_popup.vi"("error in (no error)"=w563) -> ("error out"=w568:errorcluster, "Cancel"=w561:bool, "Output Line Command"=w567:string)  [unwired: 7 in]
                n206 = Bundle By Name(cluster=w564, "Signal"=w561, "Command"=w567, "Add or modification"=TRUE) -> (w566:T2)
                n207 = case shown="True" w561 {
                  tunnel: w569 -> [w573 _]
                  tunnel: w568 -> [w572 w574]
                  tunnel: w566 -> [w571 _]
                  tunnel: [w570 w574] -> w565
                  frame False {
                    n208 = Generate User Event(user event=w573, event data cluster=w571, error in=w572) -> (error out=w570:errorcluster)  [unwired: 1 in, 1 out]
                  }
                  frame True {
                  }
                }
              }
              frame "Wait for Temperature" {
                n209 = call "SetWaitForTemp_popup.vi"("error in (no error)"=w577) -> ("Output Line Command"=w581:string, "Cancel"=w575:bool, "error out"=w582:errorcluster)  [unwired: 7 in]
                n210 = Bundle By Name(cluster=w578, "Signal"=w575, "Command"=w581, "Add or modification"=TRUE) -> (w580:T2)
                n211 = case shown="True" w575 {
                  tunnel: w583 -> [w587 _]
                  tunnel: w582 -> [w586 w588]
                  tunnel: w580 -> [w585 _]
                  tunnel: [w584 w588] -> w579
                  frame False {
                    n212 = Generate User Event(user event=w587, event data cluster=w585, error in=w586) -> (error out=w584:errorcluster)  [unwired: 1 in, 1 out]
                  }
                  frame True {
                  }
                }
              }
              frame "Wait for" {
                n213 = call "SetWaitFor_popup.vi"("error in (no error)"=w591) -> ("error out"=w596:errorcluster, "Cancel"=w589:bool, "Output Line Command"=w595:string)  [unwired: 7 in]
                n214 = Bundle By Name(cluster=w592, "Signal"=w589, "Command"=w595, "Add or modification"=TRUE) -> (w594:T2)
                n215 = case shown="False" w589 {
                  tunnel: w597 -> [w601 _]
                  tunnel: w596 -> [w600 w602]
                  tunnel: w594 -> [w599 _]
                  tunnel: [w598 w602] -> w593
                  frame False {
                    n216 = Generate User Event(user event=w601, event data cluster=w599, error in=w600) -> (error out=w598:errorcluster)  [unwired: 1 in, 1 out]
                  }
                  frame True {
                  }
                }
              }
              frame "Start" {
                n217 = call "SetStart_popup.vi"("error in (no error)"=w605) -> ("Output Line Command"=w609:string, "Cancel"=w603:bool, "error out"=w610:errorcluster)  [unwired: 7 in]
                n218 = Bundle By Name(cluster=w606, "Signal"=w603, "Command"=w609, "Add or modification"=TRUE) -> (w608:T2)
                n219 = case shown="True" w603 {
                  tunnel: w611 -> [w615 _]
                  tunnel: w610 -> [w614 w616]
                  tunnel: w608 -> [w613 _]
                  tunnel: [w612 w616] -> w607
                  frame False {
                    n220 = Generate User Event(user event=w615, event data cluster=w613, error in=w614) -> (error out=w612:errorcluster)  [unwired: 1 in, 1 out]
                  }
                  frame True {
                  }
                }
              }
              frame "Remarks" {
                n221 = call "SetRemarks_popup.vi"("error in (no error)"=w619) -> ("Cancel"=w617:bool, "Output Line Command"=w623:string, "error out"=w624:errorcluster)  [unwired: 7 in]
                n222 = Bundle By Name(cluster=w620, "Signal"=w617, "Command"=w623, "Add or modification"=TRUE) -> (w622:T2)
                n223 = case shown="True" w617 {
                  tunnel: w625 -> [w629 _]
                  tunnel: w624 -> [w628 w630]
                  tunnel: w622 -> [w627 _]
                  tunnel: [w626 w630] -> w621
                  frame False {
                    n224 = Generate User Event(user event=w629, event data cluster=w627, error in=w628) -> (error out=w626:errorcluster)  [unwired: 1 in, 1 out]
                  }
                  frame True {
                  }
                }
              }
              frame "Run Sequence" {
                n225 = call "SetRunSeq_popup.vi"("error in (no error)"=w633) -> ("error out"=w638:errorcluster, "Output Line Command"=w637:string, "Cancel"=w631:bool)  [unwired: 8 in]
                n226 = Bundle By Name(cluster=w634, "Signal"=w631, "Command"=w637, "Add or modification"=TRUE) -> (w636:T2)
                n227 = case shown="True" w631 {
                  tunnel: w639 -> [w643 _]
                  tunnel: w638 -> [w642 w644]
                  tunnel: w636 -> [w641 _]
                  tunnel: [w640 w644] -> w635
                  frame False {
                    n228 = Generate User Event(user event=w643, event data cluster=w641, error in=w642) -> (error out=w640:errorcluster)  [unwired: 1 in, 1 out]
                  }
                  frame True {
                  }
                }
              }
              frame "Run VI" {
                n229 = call "SetRunVI_popup.vi"("error in (no error)"=w647) -> ("Cancel"=w645:bool, "Output Line Command"=w651:string, "error out"=w652:errorcluster)  [unwired: 7 in]
                n230 = Bundle By Name(cluster=w648, "Signal"=w645, "Command"=w651, "Add or modification"=TRUE) -> (w650:T2)
                n231 = case shown="True" w645 {
                  tunnel: w653 -> [w657 _]
                  tunnel: w652 -> [w656 w658]
                  tunnel: w650 -> [w655 _]
                  tunnel: [w654 w658] -> w649
                  frame False {
                    n232 = Generate User Event(user event=w657, event data cluster=w655, error in=w656) -> (error out=w654:errorcluster)  [unwired: 1 in, 1 out]
                  }
                  frame True {
                  }
                }
              }
              frame "Abort VI" {
                n233 = call "SetAbortVI_popup.vi"("error in (no error)"=w661) -> ("Cancel"=w659:bool, "Output Line Command"=w665:string, "error out"=w666:errorcluster)  [unwired: 7 in]
                n234 = Bundle By Name(cluster=w662, "Signal"=w659, "Command"=w665, "Add or modification"=TRUE) -> (w664:T2)
                n235 = case shown="True" w659 {
                  tunnel: w667 -> [w671 _]
                  tunnel: w666 -> [w670 w672]
                  tunnel: w664 -> [w669 _]
                  tunnel: [w668 w672] -> w663
                  frame False {
                    n236 = Generate User Event(user event=w671, event data cluster=w669, error in=w670) -> (error out=w668:errorcluster)  [unwired: 1 in, 1 out]
                  }
                  frame True {
                  }
                }
              }
              frame "Set Parameter" {
                n237 = call "SetParameter_popup.vi"("error in (no error)"=w675) -> ("error out"=w680:errorcluster, "Cancel"=w673:bool, "Output Line Command"=w679:string)  [unwired: 7 in]
                n238 = Bundle By Name(cluster=w676, "Signal"=w673, "Command"=w679, "Add or modification"=TRUE) -> (w678:T2)
                n239 = case shown="False" w673 {
                  tunnel: w681 -> [w685 _]
                  tunnel: w680 -> [w684 w686]
                  tunnel: w678 -> [w683 _]
                  tunnel: [w682 w686] -> w677
                  frame False {
                    n240 = Generate User Event(user event=w685, event data cluster=w683, error in=w684) -> (error out=w682:errorcluster)  [unwired: 1 in, 1 out]
                  }
                  frame True {
                  }
                }
              }
              frame "Write to VISA instrument" {
                n241 = call "WriteVISA_popup.vi"("error in (no error)"=w689) -> ("Output Line Command"=w693:string, "Cancel"=w687:bool, "error out"=w694:errorcluster)  [unwired: 8 in]
                n242 = Bundle By Name(cluster=w690, "Signal"=w687, "Command"=w693, "Add or modification"=TRUE) -> (w692:T2)
                n243 = case shown="False" w687 {
                  tunnel: w695 -> [w699 _]
                  tunnel: w694 -> [w698 w700]
                  tunnel: w692 -> [w697 _]
                  tunnel: [w696 w700] -> w691
                  frame False {
                    n244 = Generate User Event(user event=w699, event data cluster=w697, error in=w698) -> (error out=w696:errorcluster)  [unwired: 1 in, 1 out]
                  }
                  frame True {
                  }
                }
              }
              frame "Set" {
                n245 = call "SetDevice_popup.vi"("error in (no error)"=w703) -> ("Cancel"=w701:bool, "Output Line Command"=w707:string, "error out"=w708:errorcluster)  [unwired: 7 in]
                n246 = Bundle By Name(cluster=w704, "Signal"=w701, "Command"=w707, "Add or modification"=TRUE) -> (w706:T2)
                n247 = case shown="True" w701 {
                  tunnel: w709 -> [w713 _]
                  tunnel: w708 -> [w712 w714]
                  tunnel: w706 -> [w711 _]
                  tunnel: [w710 w714] -> w705
                  frame False {
                    n248 = Generate User Event(user event=w713, event data cluster=w711, error in=w712) -> (error out=w710:errorcluster)  [unwired: 1 in, 1 out]
                  }
                  frame True {
                  }
                }
              }
              frame "Sweep" {
                n249 = call "SetSweep_popup.vi"("error in (no error)"=w717) -> ("Cancel"=w715:bool, "Output Line Command"=w721:string, "error out"=w722:errorcluster)  [unwired: 7 in]
                n250 = Bundle By Name(cluster=w718, "Signal"=w715, "Command"=w721, "Add or modification"=TRUE) -> (w720:T2)
                n251 = case shown="True" w715 {
                  tunnel: w723 -> [w727 _]
                  tunnel: w722 -> [w726 w728]
                  tunnel: w720 -> [w725 _]
                  tunnel: [w724 w728] -> w719
                  frame False {
                    n252 = Generate User Event(user event=w727, event data cluster=w725, error in=w726) -> (error out=w724:errorcluster)  [unwired: 1 in, 1 out]
                  }
                  frame True {
                  }
                }
              }
              frame "Stop" {
                w729 = FALSE ("Signal")
                n253 = Bundle By Name(cluster=w733, "Signal"=w729, "Command"="Stop", "Add or modification"=TRUE) -> (w735:T2)
                n254 = case shown="False" w729 {
                  tunnel: w736 -> [w740 _]
                  tunnel: w735 -> [w739 _]
                  tunnel: [w738 w741] -> w734
                  tunnel: w730 -> [w737 w741]
                  frame False {
                    n255 = Generate User Event(user event=w740, event data cluster=w739, error in=w737) -> (error out=w738:errorcluster)  [unwired: 1 in, 1 out]
                  }
                  frame True {
                  }
                }
              }
              frame "Wait for Field Stable" {
                w742 = FALSE ("Signal")
                n256 = Bundle By Name(cluster=w747, "Signal"=w742, "Command"="Wait for Field Stable", "Add or modification"=TRUE) -> (w743:T2)
                n257 = case shown="True" w742 {
                  tunnel: w749 -> [w753 _]
                  tunnel: w743 -> [w752 _]
                  tunnel: [w751 w754] -> w748
                  tunnel: w744 -> [w750 w754]
                  frame False {
                    n258 = Generate User Event(user event=w753, event data cluster=w752, error in=w750) -> (error out=w751:errorcluster)  [unwired: 1 in, 1 out]
                  }
                  frame True {
                  }
                }
              }
              frame "Wait for VI value" {
                n259 = call "SetWaitForAnyVI_popup.vi"("error in (no error)"=w759) -> ("error out"=w755:errorcluster, "Cancel"=w756:bool, "Output Line Command"=w758:string)  [unwired: 7 in]
                n260 = Bundle By Name(cluster=w761, "Signal"=w756, "Command"=w758, "Add or modification"=TRUE ("Signal")) -> (w760:T2)
                n261 = case shown="False" w756 {
                  tunnel: w763 -> [w767 _]
                  tunnel: w760 -> [w766 _]
                  tunnel: [w765 w768] -> w762
                  tunnel: w755 -> [w764 w768]
                  frame False {
                    n262 = Generate User Event(user event=w767, event data cluster=w766, error in=w764) -> (error out=w765:errorcluster)  [unwired: 1 in, 1 out]
                  }
                  frame True {
                  }
                }
              }
              frame "Run Macro" {
                n263 = call "RunMacro_popup.vi"("load?"=FALSE, "platform"=w769, "error in (no error)"=w775) -> ("Cancel"=w771:bool, "command out"=w772:string, "error out"=w773:errorcluster)  [unwired: 5 in]
                n264 = Bundle By Name(cluster=w777, "Signal"=w771, "Command"=w772, "Add or modification"=TRUE ("Signal")) -> (w776:T2)
                n265 = case shown="False" w771 {
                  tunnel: w779 -> [w783 _]
                  tunnel: w776 -> [w782 _]
                  tunnel: [w781 w784] -> w778
                  tunnel: w773 -> [w780 w784]
                  frame False {
                    n266 = Generate User Event(user event=w783, event data cluster=w782, error in=w780) -> (error out=w781:errorcluster)  [unwired: 1 in, 1 out]
                  }
                  frame True {
                  }
                }
              }
            }
          }
          event "Sequence": Double Click {
            # "check if the sequence is changed.\n(1) 'cancel' button pressed \nOR (2) no value is changed"
            n267 = event-data() -> ("Row"=w798:i32)  [unwired: 1 in]
            n268 = Unbundle By Name(w797) -> ("Sequence Reference"=w802:refnum<vi>)
            n269 = Bundle By Name(cluster=w807, "No. of line"=w798) -> (w806:T1)
            n270 = call "Library2.vi"("Message_command_in"=w806, "error in (no error)"=w805) -> ("Message_command out"=w804:T3, "error out"=w801:errorcluster)  [unwired: 7 in]
            n271 = property class="LstBox (strict)"(reference=w802, error in=w801) -> (error out=w800:errorcluster, "Item Names"=w799:string[])  [unwired: 1 out]
            n272 = Unbundle By Name(w804) -> ("No. of command"=w803:i32)
            n273 = Index Array(array=w799, index=w798) -> (element=w790:string)
            n274 = case shown="15" w803 {
              tunnel: w800 -> [w823 w830 w837 w844 w851 w858 w867 w874 w881 w888 w895 w902 w909 w916 w920]
              tunnel: w790 -> [w822 w829 w836 w843 w850 w856 w866 w873 w880 w887 w894 w901 w908 w915 _]
              tunnel: w797 -> [w820 w827 w834 w841 w848 w860 w864 w871 w878 w885 w892 w899 w905 w913 w919]
              tunnel: w796 -> [w819 w826 w833 w840 w847 w859 w863 w870 w877 w884 w891 w898 w904 w912 w918]
              tunnel: [w821 w828 w835 w842 w849 w857 w865 w872 w879 w886 w893 w900 w906 w914 w920] -> w793
              tunnel: [w820 w827 w834 w841 w848 w860 w864 w871 w878 w885 w892 w899 w905 w913 w919] -> w795
              tunnel: [w819 w826 w833 w840 w847 w859 w863 w870 w877 w884 w891 w898 w904 w912 w918] -> w794
              tunnel: [w818 w825 w832 w839 w846 w854 w862 w869 w876 w883 w889 w896 w903 w910 TRUE ("Cancel")] -> w787
              tunnel: [w817 w824 w831 w838 w845 w853 w861 w868 w875 w882 w890 w897 w907 w911 _] -> w789
              tunnel: w785 -> [_ _ _ _ _ w852 _ _ _ _ _ _ _ _ _]
              frame 0 {
                n275 = call "SetField_popup.vi"("error in (no error)"=w823, "Input Line command"=w822) -> ("Output Line command"=w817:string, "Cancel"=w818:bool, "error out"=w821:errorcluster)  [unwired: 4 in]
              }
              frame 1 {
                n276 = call "SetTemp_popup.vi"("Input Line Command"=w829, "error in (no error)"=w830) -> ("error out"=w828:errorcluster, "Cancel"=w825:bool, "Output Line Command"=w824:string)  [unwired: 6 in]
              }
              frame 2 {
                n277 = call "SetStart_popup.vi"("Input Line Command"=w836, "error in (no error)"=w837) -> ("Output Line Command"=w831:string, "Cancel"=w832:bool, "error out"=w835:errorcluster)  [unwired: 6 in]
              }
              frame 4 {
                n278 = call "SetWaitForTemp_popup.vi"("Input Line Command"=w843, "error in (no error)"=w844) -> ("Output Line Command"=w838:string, "Cancel"=w839:bool, "error out"=w842:errorcluster)  [unwired: 6 in]
              }
              frame 7 {
                n279 = call "SetRemarks_popup.vi"("Input Line Command"=w850, "error in (no error)"=w851) -> ("Cancel"=w846:bool, "Output Line Command"=w845:string, "error out"=w849:errorcluster)  [unwired: 6 in]
              }
              frame 8 {
                n280 = call "RunMacro_popup.vi"("load?"=TRUE, "platform"=w852, "command in"=w856, "error in (no error)"=w858) -> ("Cancel"=w854:bool, "command out"=w853:string, "error out"=w857:errorcluster)  [unwired: 4 in]
              }
              frame 9 {
                n281 = call "SetRunVI_popup.vi"("Input Line Command"=w866, "error in (no error)"=w867) -> ("Cancel"=w862:bool, "Output Line Command"=w861:string, "error out"=w865:errorcluster)  [unwired: 6 in]
              }
              frame 10 {
                n282 = call "SetAbortVI_popup.vi"("Input Line Command"=w873, "error in (no error)"=w874) -> ("Cancel"=w869:bool, "Output Line Command"=w868:string, "error out"=w872:errorcluster)  [unwired: 6 in]
              }
              frame 11 {
                n283 = call "SetDevice_popup.vi"("Input Line Command"=w880, "error in (no error)"=w881) -> ("Cancel"=w876:bool, "Output Line Command"=w875:string, "error out"=w879:errorcluster)  [unwired: 6 in]
              }
              frame 16 {
                n284 = call "SetSweep_popup.vi"("Input Line Command"=w887, "error in (no error)"=w888) -> ("Cancel"=w883:bool, "Output Line Command"=w882:string, "error out"=w886:errorcluster)  [unwired: 6 in]
              }
              frame 12 {
                n285 = call "SetWaitFor_popup.vi"("Input Line Command"=w894, "error in (no error)"=w895) -> ("error out"=w893:errorcluster, "Cancel"=w889:bool, "Output Line Command"=w890:string)  [unwired: 6 in]
              }
              frame 13 {
                n286 = call "SetParameter_popup.vi"("Input Line Command"=w901, "error in (no error)"=w902) -> ("error out"=w900:errorcluster, "Cancel"=w896:bool, "Output Line Command"=w897:string)  [unwired: 6 in]
              }
              frame 14 {
                n287 = call "SetWaitForAnyVI_popup.vi"("Input Line Command"=w908, "error in (no error)"=w909) -> ("error out"=w906:errorcluster, "Cancel"=w903:bool, "Output Line Command"=w907:string)  [unwired: 6 in]
              }
              frame 15 {
                n288 = call "WriteVISA_popup.vi"("error in (no error)"=w916, "Input Line Command"=w915) -> ("Output Line Command"=w911:string, "Cancel"=w910:bool, "error out"=w914:errorcluster)  [unwired: 7 in]
              }
              frame Default {
              }
            }
            n289 = Equal?(x=w790, y=w789) -> (x = y?=w788:bool)
            n290 = Or(x=w787, y=w788) -> (x .or. y?=w786:bool)
            n291 = case shown="False" w786 {
              selector: w786 -> [w810 _]
              tunnel: w795 -> [w814 _]
              tunnel: w794 -> [w812 _]
              tunnel: w789 -> [w811 _]
              tunnel: w793 -> [w809 w816]
              tunnel: [w808 w816] -> w792
              frame False {
                n292 = Bundle By Name(cluster=w814, "Signal"=w810, "Command"=w811, "Add or modification"=FALSE) -> (w813:T2)
                n293 = Generate User Event(user event=w812, event data cluster=w813, error in=w809) -> (error out=w808:errorcluster)  [unwired: 1 in, 1 out]
              }
              frame True {
              }
            }
          }
          event "Sequence": Value Change {
            n294 = event-data() -> ("NewVal"=w925:i32[])  [unwired: 1 in]
            n295 = Index Array(array=w925, index=0) -> (element=→"Cursor Position":i32)
          }
          event "OK Button": Value Change {
            # "Press OK button saves the sequence and exit"
            n296 = event-data() -> ()  [unwired: 1 in, 6 out]
            n297 = property on="Path" class="Path"(error in=w929) -> (error out=w931:errorcluster, "Value"=w936:path)  [unwired: 1 in, 1 out]
            n298 = property on="Buffer History" class="Arr (strict)"(error in=w931) -> (error out=w932:errorcluster, "Value"=w933:string[])  [unwired: 1 in, 1 out]
            n299 = Not Equal?(x=path "", y=w936) -> (x != y?=w937:bool)
            n300 = property on="Sequence" class="LstBox (strict)"(error in=w932) -> ("Item Names"=w934:string[], "Caption.Text"=w935:string)  [unwired: 1 in, 2 out]
            n301 = call "Save_File.vi"("Sequence caption in"=w935, "Path?"=w937, "Sequence in"=w934, "Buffer in"=w933, "Path in"=w936) -> ("error out"=w941:errorcluster, "Sequence out"=w938:string[], "Buffer out"=w939:string[], "Path out"=w927:path, "Sequence caption out"=w942:string)  [unwired: 2 in]
            n302 = property on="Buffer History" class="Arr (strict)"(error in=w941, "Value"=w939) -> (error out=w940:errorcluster)  [unwired: 1 in, 1 out]
            n303 = property on="Sequence" class="LstBox (strict)"(error in=w940, "Item Names"=w938, "Caption.Text"=w942) -> (error out=w943:errorcluster)  [unwired: 1 in, 1 out]
            n304 = property on="Path" class="Path"(error in=w943, "Value"=w927) -> (error out=w928:errorcluster)  [unwired: 1 in, 1 out]
            n305 = Path To String(path=w927) -> (string=w946:string)
            n306 = Concatenate Strings("Run Macro " ("string"), w946) -> (→"command out":string)
            n307 = property on="Cancel" class="Bool (strict)"(error in=w928, "Value"=FALSE ("Cancel")) -> (error out=w945:errorcluster)  [unwired: 1 in, 1 out]
          }
          event "Cancel Button": Value Change {
            # "Press Cancel button \nFor existing sequence command: revert  the sequence (by saving initially loaded sequnece)\nand exit.\nFor new command : nothing happends and exit"
            n308 = event-data() -> ()  [unwired: 1 in, 6 out]
            n309 = case shown="False" w953 {
              tunnel: w952 -> [_ w963]
              tunnel: w951 -> [_ w962]
              tunnel: w950 -> [w957 w960]
              tunnel: [w957 w958] -> w949
              frame False {
              }
              frame True {
                n310 = Path To String(path=w963) -> (string=w966:string)
                n311 = call "Save_File.vi"("Sequence caption in"="Sequence" ("Caption.Text"), "Path?"=TRUE, "error in (no error)"=w960, "Sequence in"=w962, "Path in"=w963) -> ("error out"=w959:errorcluster)  [unwired: 2 in, 4 out]
                n312 = Concatenate Strings("Run Macro " ("string"), w966) -> (w965:string)
                n313 = property on="command out" class="Str"(error in=w959, "Value"=w965) -> (error out=w958:errorcluster)  [unwired: 1 in, 1 out]
              }
            }
            n314 = property on="Cancel" class="Bool (strict)"(error in=w949, "Value"=TRUE ("Cancel")) -> (error out=w955:errorcluster)  [unwired: 1 in, 1 out]
          }
        }
      }
    }
    frame Error {
    }
  }
  n315 = Unregister For Events(event registration refnum=w27, error in=w26) -> (error out=→"error out":errorcluster)
  "Buffer History" <- w20
  "Buffer Edit" <- w20
